vi "SPD.Config Read Test06 AP.vi"(8 "Error In":errorcluster, 11 "SPD.Stand Ctrl in":T2 {"spdDeviceSession"."hidSPD.Sturtup Values"."HV_bias" format="%#_6p, V"; "spdDeviceSession"."hidSPD.Sturtup Values"."TSet" format="%#_6p, DegC"; "spdDeviceSession"."hidSPD.Controller"."HV_bias" format="%#_6p, V"; "spdDeviceSession"."hidSPD.Controller"."TSet" format="%#_6p, DegC"}) -> (0 "Error Out":errorcluster, 2 "AP Meas Params":T1, 3 "SPD.Stand Ctrl out":T2 {"spdDeviceSession"."hidSPD.Sturtup Values"."HV_bias" format="%#_6p, V"; "spdDeviceSession"."hidSPD.Sturtup Values"."TSet" format="%#_6p, DegC"; "spdDeviceSession"."hidSPD.Controller"."HV_bias" format="%#_6p, V"; "spdDeviceSession"."hidSPD.Controller"."TSet" format="%#_6p, DegC"})   [LabVIEW 2018]
uses:
  typedefs/SPD.Stand Ctrl.ctl
  Instruments/SPD HID Interface/hidSPDLibForLabView/LibVIs/hidSPD Controls/hidSPD Device Session.ctl
  Instruments/SPD HID Interface/hidSPDLibForLabView/LibVIs/hidSPD Controls/hidSPD Controller.ctl
  Instruments/SPD HID Interface/hidSPDLibForLabView/LibVIs/hidSPD Controls/hidSPD SPD Type.ctl
  Instruments/KC705 DevBoard/typedefs/DevB.Session.ctl
  Instruments/KeySight 53230A/typedefs/FreqC.Session.ctl
  Instruments/KeySight 8164B/KeySight 8164B LAN InstrLib/typedefs/KeySight 8164B control.ctl
  Instruments/LeCroy SDA830/typedefs/LeCroy.Session.ctl
  typedefs/SPD.Events.ctl
  SPD.Config File ctrl.ctl
  <vilib>/Utility/config.llb/Config Data RefNum.ctl
  typedefs/SPD.Meas Result.ctl
  typedefs/SPD.Queues.ctl
  typedefs/SPD.Stand state.ctl
  SPD Measurements/AP/typedefs/SPD.AP Test Params.ctl
  <vilib>/Utility/config.llb/Read Key (I32).vi
  <vilib>/Utility/config.llb/Read Key (Double).vi
  <vilib>/Utility/config.llb/Read Key (String).vi
  <vilib>/Utility/config.llb/NI_LVConfig.lvlib
  Instruments/KeySight 8164B/KeySight 8164B LAN InstrLib.lvlib
  Instruments/SPD HID Interface/hidSPDLibForLabView/hidSPDLibForLabView.lvlib
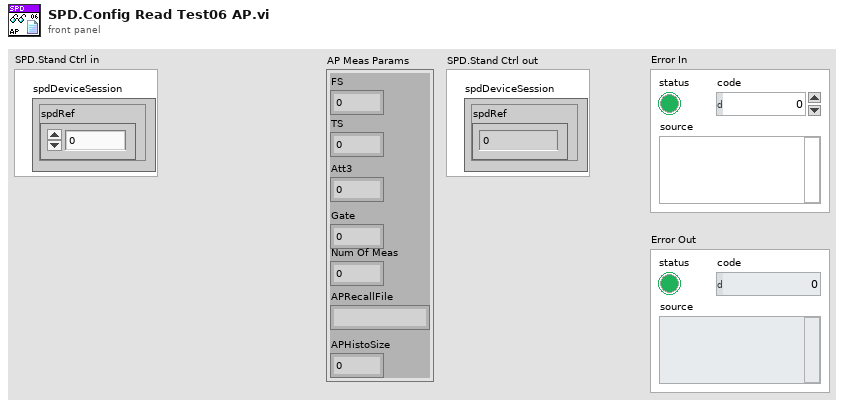
[diagram p1: front panel]
types:
  T1 = typedef "SPD.AP Test Params.ctl" = cluster{"FS":i32, "TS":i32, "Att3":dbl, "Gate":dbl, "Num Of Meas":i32, "APRecallFile":string, "APHistoSize":i32}
  T2 = typedef "SPD.Stand Ctrl.ctl" = cluster{"spdDeviceSession":T3, "DevBSession":T6, "FreqCSession":T7, "8164BSession":T8, "LeCroySession":T9, "Events":T10, "configFile":T11, "SPD.Result":T13, "SPD.Queues":T14, "Console":refnum<vi>}
  T3 = typedef "hidSPDLibForLabView.lvlib/hidSPD Device Session.ctl" = cluster{"spdRef":u64, "connected":bool, "spdName":string, "hidSPD.Controller":T4, "hidSPD.Sturtup Values":T4, "SPD Type":T5}
  T4 = typedef "hidSPDLibForLabView.lvlib/hidSPD Controller.ctl" = cluster{"TSet":sgl, "HV_bias":sgl, "DDS_stb_code":u16}
  T5 = typedef "hidSPDLibForLabView.lvlib/hidSPD SPD Type.ctl" = enum16{"Free Run", "Gate"}
  T6 = typedef "DevB.Session.ctl" = cluster{"DevBRef":refnum<visa-resource-name>, "connected":bool}
  T7 = typedef "FreqC.Session.ctl" = cluster{"FreqCRef":refnum<visa-resource-name>, "timeout":dbl, "Gate":dbl, "connected":bool}
  T8 = typedef "KeySight 8164B LAN InstrLib.lvlib/KeySight 8164B control.ctl" = cluster{"Connection ID":refnum<k5>, "Connected":bool, "Info":string, "Slots Info":string[]}
  T9 = typedef "LeCroy.Session.ctl" = cluster{"LeCroySession":refnum<visa-resource-name>, "connected":bool}
  T10 = typedef "SPD.Events.ctl" = cluster{"DCRTest":refnum<user-event>, "Stop":refnum<user-event>}
  T11 = typedef "SPD.Config File ctrl.ctl" = cluster{"configFile ref":T12, "configFile path":path, "equipmentFile ref":T12}
  T12 = typedef "NI_LVConfig.lvlib/Config Data RefNum.ctl" = refnum<k1>
  T13 = typedef "SPD.Meas Result.ctl" = cluster{"HV_Bias":dbl[][][], "Stb_code":dbl[], "Temprature":dbl[], "Data":dbl[][][][], "DateTime":string}
  T14 = typedef "SPD.Queues.ctl" = cluster{"state queue":refnum<queue>}
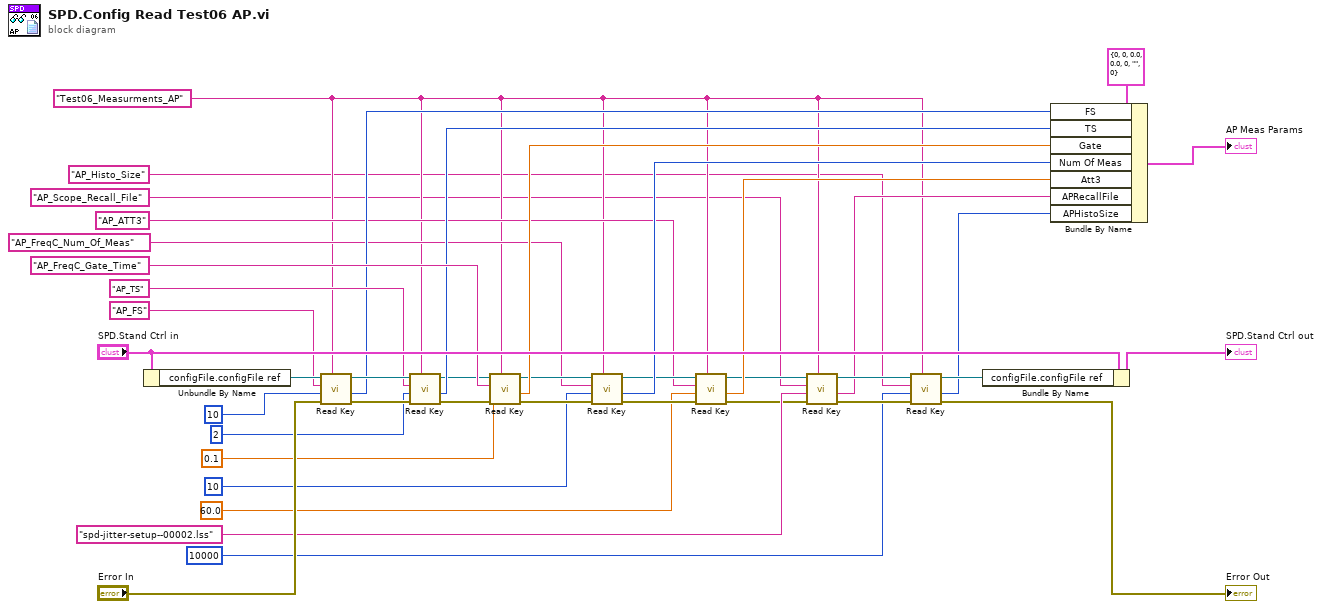
[diagram p0: block diagram]
diagram:
  w3 = "Test06_Measurments_AP" ("section")
  n1 = Unbundle By Name("SPD.Stand Ctrl in") -> ("configFile.configFile ref"=w40:T12)
  n2 = call-poly <vilib>:"Read Key.vi"("section"=w3, "error in (no error)"="Error In", "default value"=10, "key"="AP_FS", "refnum"=w40) -> ("error out"=w36:errorcluster, "value"=w30:i32, "refnum out"=w35:T12)  [unwired: 3 in, 1 out]
  n3 = call-poly <vilib>:"Read Key.vi"("section"=w3, "error in (no error)"=w36, "default value"=2, "key"="AP_TS", "refnum"=w35) -> ("error out"=w20:errorcluster, "value"=w29:i32, "refnum out"=w21:T12)  [unwired: 3 in, 1 out]
  n4 = call-poly <vilib>:"Read Key.vi"("section"=w3, "error in (no error)"=w20, "default value"=0.1, "key"="AP_FreqC_Gate_Time", "refnum"=w21) -> ("error out"=w25:errorcluster, "value"=w28:dbl, "refnum out"=w26:T12)  [unwired: 3 in, 1 out]
  n5 = call-poly <vilib>:"Read Key.vi"("section"=w3, "error in (no error)"=w25, "default value"=10, "key"="AP_FreqC_Num_Of_Meas", "refnum"=w26) -> ("error out"=w17:errorcluster, "value"=w24:i32, "refnum out"=w18:T12)  [unwired: 3 in, 1 out]
  n6 = call-poly <vilib>:"Read Key.vi"("section"=w3, "error in (no error)"=w17, "default value"=60.0, "key"="AP_ATT3", "refnum"=w18) -> ("error out"=w4:errorcluster, "value"=w14:dbl, "refnum out"=w5:T12)  [unwired: 3 in, 1 out]
  n7 = call-poly <vilib>:"Read Key.vi"("section"=w3, "error in (no error)"=w4, "default value"="spd-jitter-setup--00002.lss", "key"="AP_Scope_Recall_File", "refnum"=w5) -> ("error out"=w12:errorcluster, "value"=w8:string, "refnum out"=w13:T12)  [unwired: 3 in, 1 out]
  n8 = call-poly <vilib>:"Read Key.vi"("section"=w3, "error in (no error)"=w12, "default value"=10000, "key"="AP_Histo_Size", "refnum"=w13) -> ("error out"=→"Error Out":errorcluster, "value"=w6:i32, "refnum out"=w11:T12)  [unwired: 3 in, 1 out]
  n9 = Bundle By Name(cluster="SPD.Stand Ctrl in", "configFile.configFile ref"=w11) -> (→"SPD.Stand Ctrl out":T2)
  n10 = Bundle By Name(cluster=T1 {"FS"=0, "TS"=0, "Att3"=0.0, "Gate"=0.0, "Num Of Meas"=0, "APRecallFile"="", "APHistoSize"=0} ("APParams"), "FS"=w30, "TS"=w29, "Gate"=w28, "Num Of Meas"=w24, "Att3"=w14, "APRecallFile"=w8, "APHistoSize"=w6) -> (→"AP Meas Params":T1)
